vi "Tencion Graph Drawer.vi"(8 "error in":errorcluster, 10 "Right Tencion":dbl[](array[numeric]), 11 "Left Tencion":dbl[](array[numeric])) -> (0 "error out":errorcluster, 3 "Tencion Graph":cluster{dbl[], dbl[]}[](graph))   [LabVIEW 2025]
uses:
  <vilib>/Analysis/baseanly.llb/Mean (DBL).vi
  <vilib>/Analysis/NI_AALBase.lvlib
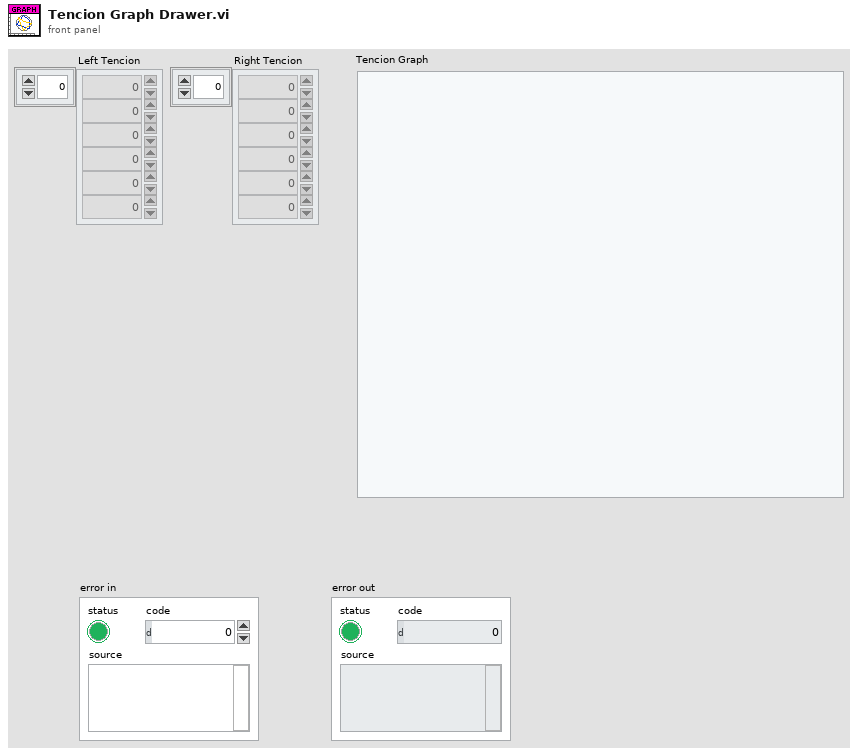
[diagram p1: front panel]
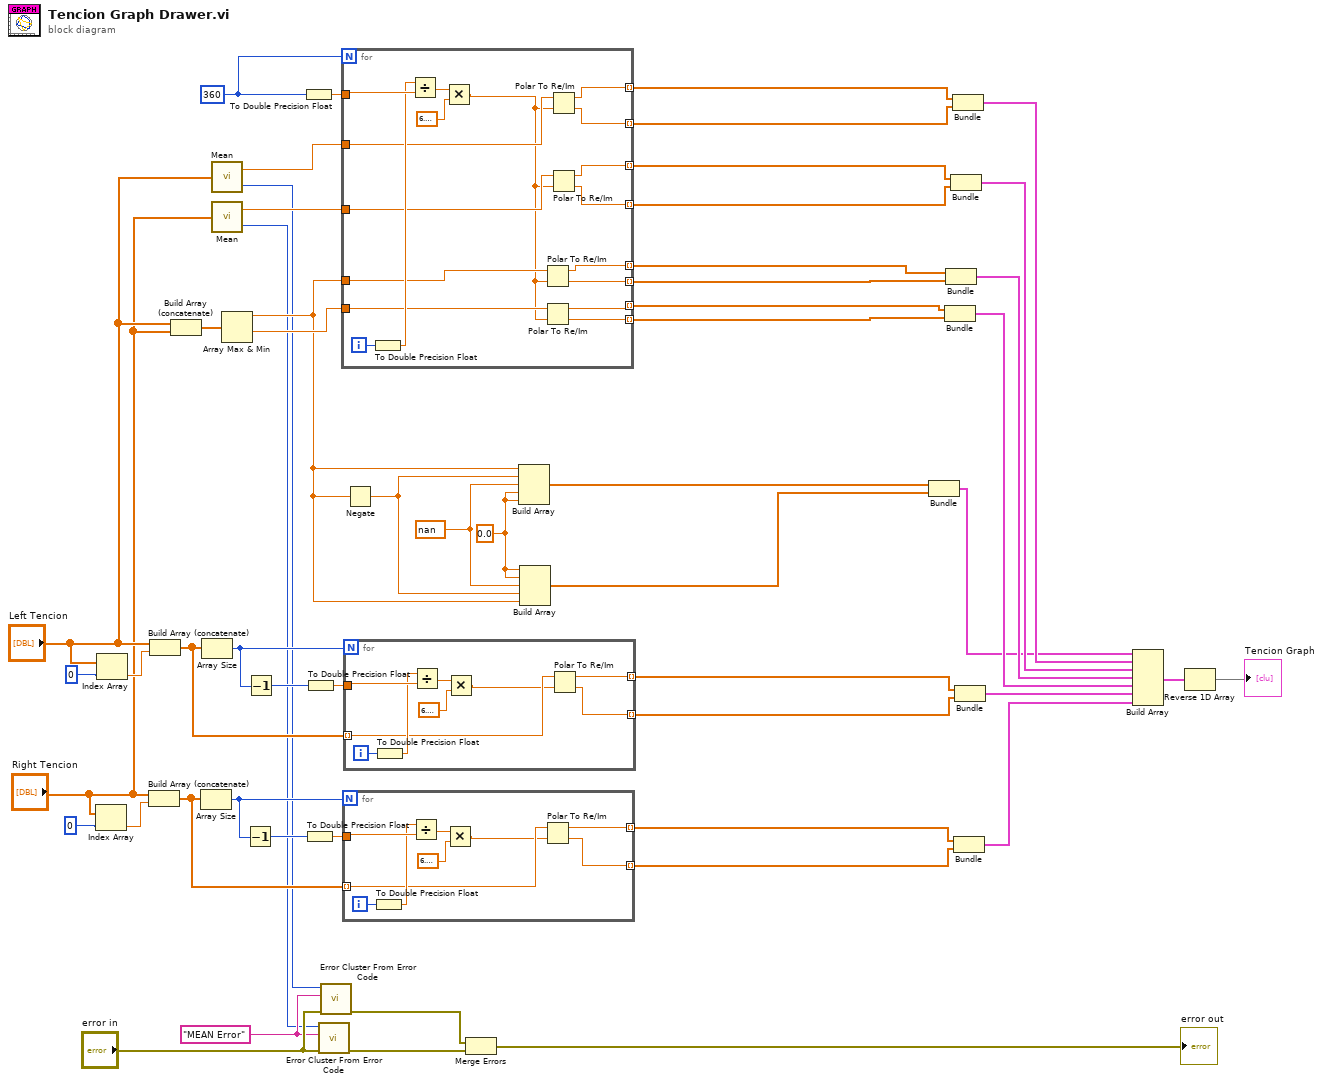
[diagram p0: block diagram]
diagram:
  w3 = "MEAN Error" ("error message (\"\")")
  w14 = 0.0 ("element")
  w15 = nan
  w33 = 360
  n1 = Index Array(array="Right Tencion", index=0) -> (element=w42:dbl)
  n2 = Index Array(array="Left Tencion", index=0) -> (element=w51:dbl)
  n3 = Build Array (concatenate)("Right Tencion", w42) -> (w40:dbl[])
  n4 = Build Array (concatenate)("Left Tencion", w51) -> (w49:dbl[])
  n5 = Build Array (concatenate)("Left Tencion", "Right Tencion") -> (w30:dbl[])
  n6 = Array Size(array=w40) -> (size(s)=w38:i32)
  n7 = Array Size(array=w49) -> (size(s)=w47:i32)
  n8 = call-poly <vilib>:"Mean.vi"("X"="Left Tencion") -> ("mean"=w8:dbl, "error"=w2:i32)
  n9 = call-poly <vilib>:"Mean.vi"("X"="Right Tencion") -> ("mean"=w9:dbl, "error"=w1:i32)
  n10 = Array Max & Min(array=w30) -> (max value=w16:dbl, min value=w27:dbl)  [unwired: 2 out]
  n11 = Decrement(x=w38) -> (x-1=w39:i32)
  n12 = Decrement(x=w47) -> (x-1=w48:i32)
  n13 = To Double Precision Float(number=w33) -> (double precision float=w36:dbl)
  n14 = To Double Precision Float(number=w39) -> (double precision float=w45:dbl)
  n15 = To Double Precision Float(number=w48) -> (double precision float=w54:dbl)
  n16 = call <vilib>:"Error Cluster From Error Code.vi"("error in (no error)"="error in", "error message (\"\")"=w3, "error code (0)"=w1) -> ("error out"=w6:errorcluster)  [unwired: 6 in]
  n17 = call <vilib>:"Error Cluster From Error Code.vi"("error in (no error)"="error in", "error message (\"\")"=w3, "error code (0)"=w2) -> ("error out"=w5:errorcluster)  [unwired: 6 in]
  n18 = for {
    N: w33 -> [_]
    tunnel: w36 -> [w69]
    tunnel: [w62] -> w34 mode=indexing
    tunnel: [w63] -> w35 mode=indexing
    tunnel: w8 -> [w64]
    tunnel: [w67] -> w32 mode=indexing
    tunnel: [w66] -> w31 mode=indexing
    tunnel: w9 -> [w65]
    tunnel: w16 -> [w60]
    tunnel: w27 -> [w61]
    tunnel: [w58] -> w25 mode=indexing
    tunnel: [w57] -> w26 mode=indexing
    tunnel: [w56] -> w24 mode=indexing
    tunnel: [w55] -> w23 mode=indexing
    i -> [w72]
    n19 = To Double Precision Float(number=w72) -> (double precision float=w68:dbl)
    n20 = Divide(x=w68, y=w69) -> (x/y=w71:dbl)
    n21 = Multiply(x=w71, y=6.283185307179586) -> (x*y=w59:dbl)
    n22 = Polar To Re/Im(2:w59, 3:w60) -> (0:w58:dbl, 1:w57:dbl)
    n23 = Polar To Re/Im(2:w59, 3:w61) -> (0:w55:dbl, 1:w56:dbl)
    n24 = Polar To Re/Im(2:w59, 3:w64) -> (0:w62:dbl, 1:w63:dbl)
    n25 = Polar To Re/Im(2:w59, 3:w65) -> (0:w66:dbl, 1:w67:dbl)
  }
  n26 = for {
    N: w38 -> [_]
    tunnel: w45 -> [w78]
    tunnel: [w75] -> w43 mode=indexing
    tunnel: [w76] -> w44 mode=indexing
    tunnel: w40 -> [w74] mode=indexing
    i -> [w81]
    n27 = To Double Precision Float(number=w81) -> (double precision float=w77:dbl)
    n28 = Divide(x=w77, y=w78) -> (x/y=w80:dbl)
    n29 = Multiply(x=w80, y=6.283185307179586) -> (x*y=w73:dbl)
    n30 = Polar To Re/Im(2:w73, 3:w74) -> (0:w75:dbl, 1:w76:dbl)
  }
  n31 = for {
    N: w47 -> [_]
    tunnel: w54 -> [w87]
    tunnel: [w82] -> w52 mode=indexing
    tunnel: [w83] -> w53 mode=indexing
    tunnel: w49 -> [w85] mode=indexing
    i -> [w90]
    n32 = To Double Precision Float(number=w90) -> (double precision float=w86:dbl)
    n33 = Divide(x=w86, y=w87) -> (x/y=w89:dbl)
    n34 = Multiply(x=w89, y=6.283185307179586) -> (x*y=w84:dbl)
    n35 = Polar To Re/Im(2:w84, 3:w85) -> (0:w82:dbl, 1:w83:dbl)
  }
  n36 = Negate(x=w16) -> (-x=w17:dbl)
  n37 = Merge Errors(w5, w6) -> (→"error out":errorcluster)
  n38 = Build Array(w16, w17, w15, w14, w14) -> (w20:dbl[])
  n39 = Build Array(w14, w14, w15, w17, w16) -> (w19:dbl[])
  n40 = Bundle(w20, w19) -> (w18:cluster{dbl[], dbl[]})  [unwired: 1 in]
  n41 = Bundle(w24, w23) -> (w22:cluster{dbl[], dbl[]})  [unwired: 1 in]
  n42 = Bundle(w26, w25) -> (w21:cluster{dbl[], dbl[]})  [unwired: 1 in]
  n43 = Bundle(w32, w31) -> (w29:cluster{dbl[], dbl[]})  [unwired: 1 in]
  n44 = Bundle(w35, w34) -> (w28:cluster{dbl[], dbl[]})  [unwired: 1 in]
  n45 = Bundle(w44, w43) -> (w37:cluster{dbl[], dbl[]})  [unwired: 1 in]
  n46 = Bundle(w53, w52) -> (w46:cluster{dbl[], dbl[]})  [unwired: 1 in]
  n47 = Build Array(w18, w28, w29, w21, w22, w46, w37) -> (w13:cluster{dbl[], dbl[]}[])
  n48 = Reverse 1D Array(array=w13) -> (reversed array=→"Tencion Graph":cluster{dbl[], dbl[]}[])
